vi "Update Data.vi"(8 "error in (no error)":errorcluster, 10 "Debug Data":refnum<class "Debug Data.lvclass">[](array[class]), 11 "List Seen Processes View Model In":refnum<class "Multicolumn List Box View Model.lvclass">) -> (0 "error out":errorcluster, 3 "List Seen Processes View Model Out":refnum<class "Multicolumn List Box View Model.lvclass">)   [LabVIEW 2020, in "Multicolumn List Box View Model.lvclass"]
uses:
  Multicolumn List Box View Model.lvclass
  Debug Data/Debug Data.lvclass
  Debug Data/Debug Data.lvclass/Debug Data.ctl
  Multicolumn List Box View Model.lvclass/Multicolumn List Box View Model.ctl
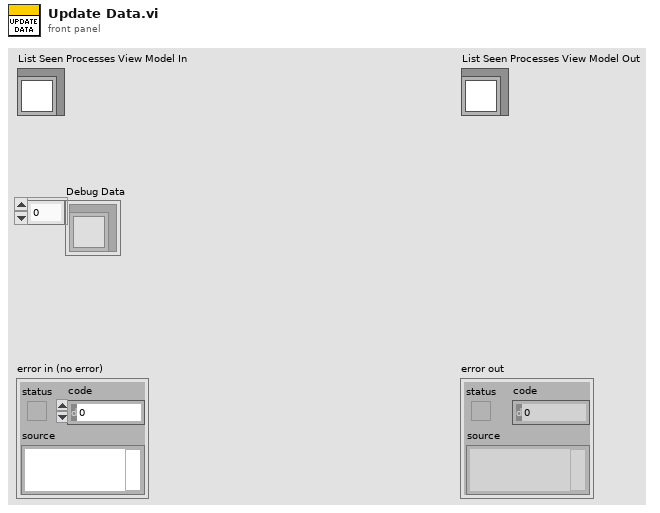
[diagram p1: front panel]
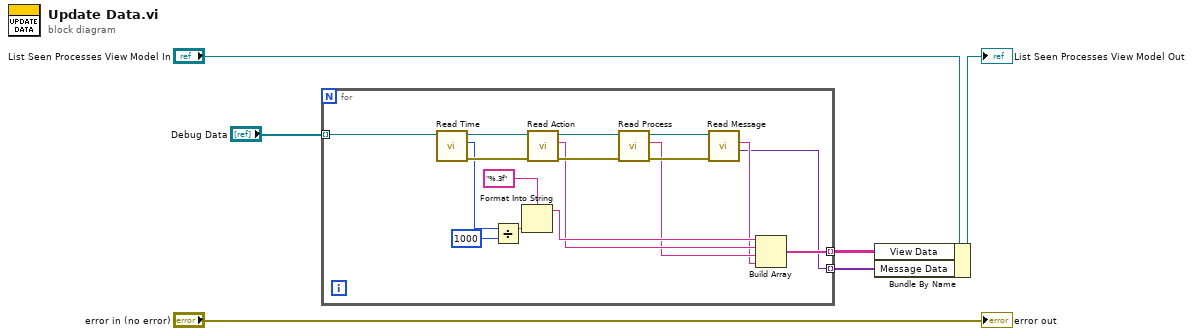
[diagram p0: block diagram]
diagram:
  n1 = for {
    tunnel: "Debug Data" -> [w20] mode=indexing
    tunnel: [w8] -> w2 mode=indexing
    tunnel: [w7] -> w1 mode=indexing
    n2 = call "Read Time.vi"("Debug Data in"=w20) -> ("error out"=w23:errorcluster, "Time"=w19:u32, "Debug Data out"=w13:refnum<class "Debug Data.lvclass">)  [unwired: 8 in]
    n3 = Divide(x=w19, y=u32 1000) -> (x/y=w18:dbl)
    n4 = Format Into String(format string="%.3f", w18) -> (resulting string=w15:string)  [unwired: 2 in, 1 out]
    n5 = call "Read Action.vi"("error in (no error)"=w23, "Debug Data in"=w13) -> ("error out"=w14:errorcluster, "Action"=w11:string, "Debug Data out"=w12:refnum<class "Debug Data.lvclass">)  [unwired: 7 in]
    n6 = call "Read Process.vi"("error in (no error)"=w14, "Debug Data In"=w12) -> ("error out"=w21:errorcluster, "Process"=w10:string, "Debug Data Out"=w22:refnum<class "Debug Data.lvclass">)  [unwired: 7 in]
    n7 = call "Read Message.vi"("error in (no error)"=w21, "Debug Data in"=w22) -> ("Message Data"=w7:variant, "Message"=w9:string)  [unwired: 6 in, 2 out]
    n8 = Build Array(w15, w11, w10, w9) -> (w8:string[])
  }
  n9 = Bundle By Name(cluster="List Seen Processes View Model In", "View Data"=w2, "Message Data"=w1) -> (→"List Seen Processes View Model Out":refnum<class "Multicolumn List Box View Model.lvclass">)
  "error out" <- "error in (no error)"
